vi "checkStatus.vi"(8 "error in (no error)":errorcluster, 10 "stop":bool, 11 "NetworkCamera in":refnum<class "NetworkCamera.lvclass">) -> (0 "error out":errorcluster, 2 "stopped?":bool, 3 "NetworkCamera out":refnum<class "NetworkCamera.lvclass">)   [LabVIEW 2009, in "Hardware.lvlib" / "HWControllers.lvlib" / "NetworkCamera.lvclass"]
uses:
  NetworkCamera.lvclass
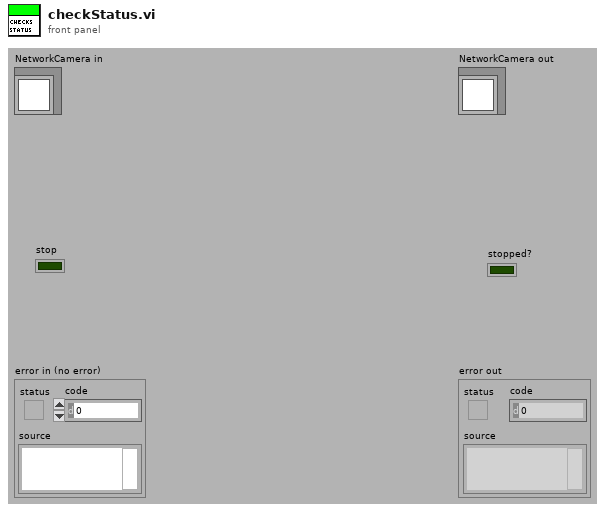
[diagram p1: front panel]
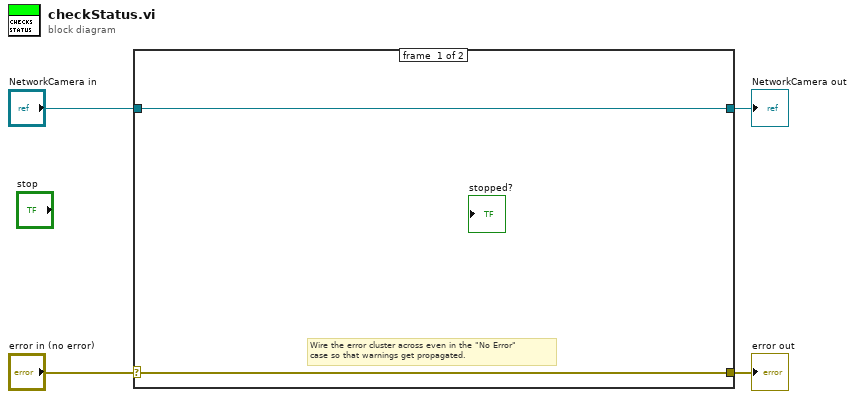
[diagram p0: block diagram]
diagram:
  n1 = case shown="No Error" "error in (no error)" {
    selector: "error in (no error)" -> [w5 w8]
    tunnel: [w5 w8] -> w3
    tunnel: [w6 w7] -> w1
    tunnel: "NetworkCamera in" -> [w6 w7]
    frame #0 {
      # "Wire the error cluster across even in the \"No Error\"\ncase so that warnings get propagated."
    }
    frame #1 {
    }
  }
  "error out" <- w3
  "NetworkCamera out" <- w1
